vi "Demo.vi"() -> ()   [LabVIEW 2013, in "GOLPI library.lvlib"]
uses:
  GOLPI library.lvlib
  LV Process.lvlibp
panel:
  in  "byte count":i32=1024
  in  "timeout [ms]":i32=10
  out "read buffer":string
  in  "write buffer":string="date /T\nexit\n"
  out "bytes written":i32
  out "exit code":i32
  out "error out":errorcluster
  in  "command":string="cmd"
  in  "working folder 2":string="c:\\"
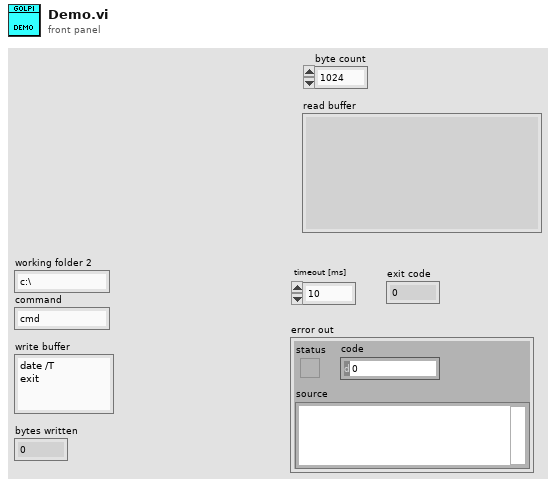
[diagram p1: front panel]
types:
  T1 = typedef "LV Process.lvlibp/Pipe Handle.ctl" = cluster{"lv_proc.dll file path":path, "process instance handle":u32[]}
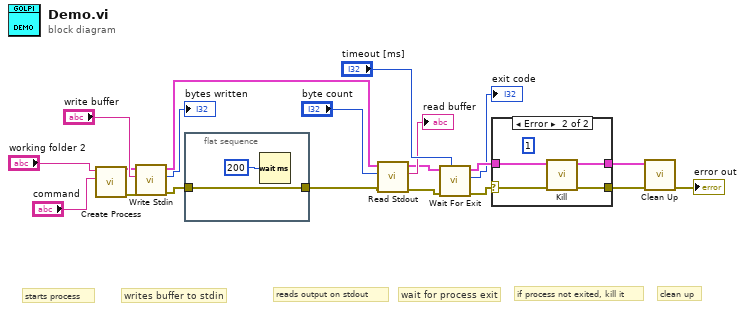
[diagram p0: block diagram]
diagram:
  # "clean up"
  # "if process not exited, kill it"
  # "wait for process exit"
  # "reads output on stdout"
  # "writes buffer to stdin"
  # "starts process"
  n1 = call "Create Process.vi"("command"="command", "working folder"="working folder 2") -> ("error out"=w20:errorcluster, "pipe handle"=w16:T1)  [unwired: 8 in]
  n2 = call "Write Stdin.vi"("error in"=w20, "write buffer"="write buffer", "pipe in"=w16) -> ("error out"=w19:errorcluster, "return count"=→"bytes written":i32, "pipe out"=w8:T1)  [unwired: 6 in]
  n3 = flat-sequence {
    tunnel: [w21] -> w9
    tunnel: w19 -> [w21]
    frame #0 {
      n4 = Wait (ms)(milliseconds to wait=u32 200) -> ()  [unwired: 1 out]
    }
  }
  n5 = call "Read Stdout.vi"("error in"=w9, "byte count"="byte count", "pipe in"=w8) -> ("error out"=w10:errorcluster, "read buffer"=→"read buffer":string, "pipe out"=w4:T1)  [unwired: 3 in, 3 out]
  n6 = call "Wait For Exit.vi"("timeout [ms]"="timeout [ms]", "error in"=w10, "pipe in"=w4) -> ("error out"=w11:errorcluster, "exit code"=→"exit code":i32, "pipe out"=w3:T1)  [unwired: 6 in]
  n7 = case shown="Error" w11 {
    selector: w11 -> [w23 w27]
    tunnel: w3 -> [w24 w26]
    tunnel: [w23 w28] -> w12
    tunnel: [w24 w25] -> w1
    frame No Error {
    }
    frame Error {
      (unwired) 1 ("timeout [ms]")
      n8 = call "Kill.vi"("error in"=w27, "pipe in"=w26) -> ("error out"=w28:errorcluster, "pipe out"=w25:T1)  [unwired: 8 in]
    }
  }
  n9 = call "Clean Up.vi"("error in"=w12, "pipe in"=w1) -> ("error out"=→"error out":errorcluster)  [unwired: 9 in]
